vi "Sort Particle Reports.vi"(1 "Report 2":T1, 2 "Report 1":T1) -> (0 "x > y?":bool)   [LabVIEW 2025]
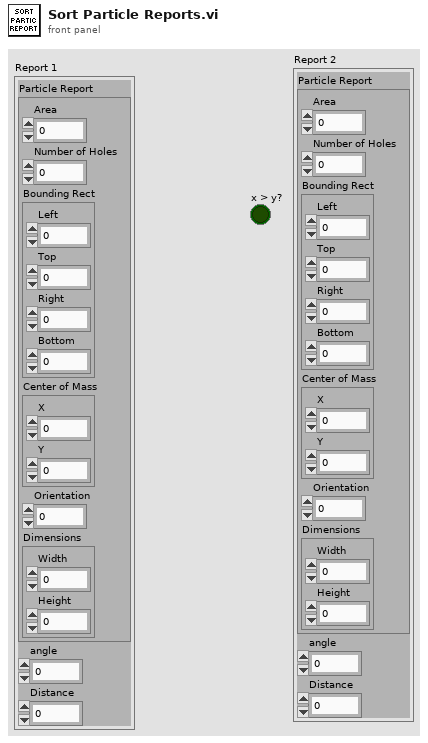
[diagram p1: front panel]
types:
  T1 = cluster{"Particle Report":cluster{"Area":dbl, "Number of Holes":dbl, "Bounding Rect":cluster{"Left":dbl, "Top":dbl, "Right":dbl, "Bottom":dbl}, "Center of Mass":cluster{"X":dbl, "Y":dbl}, "Orientation":dbl, "Dimensions":cluster{"Width":dbl, "Height":dbl}}, "angle":dbl, "Distance":ext}
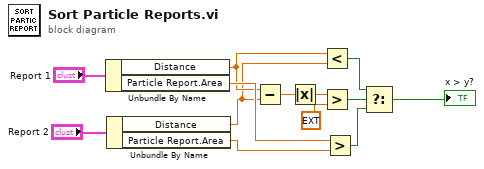
[diagram p0: block diagram]
diagram:
  n1 = Unbundle By Name("Report 1") -> ("Distance"=w3:ext, "Particle Report.Area"=w6:dbl)
  n2 = Unbundle By Name("Report 2") -> ("Distance"=w2:ext, "Particle Report.Area"=w5:dbl)
  n3 = Subtract(x=w3, y=w2) -> (x-y=w12:ext)
  n4 = Absolute Value(x=w12) -> (abs(x)=w4:ext)
  n5 = Less?(x=w3, y=w2) -> (x < y?=w1:bool)
  n6 = Greater?(x=w4, y=ext 2.0) -> (0:w11:bool)
  n7 = Greater?(x=w6, y=w5) -> (0:w7:bool)
  n8 = Select(t=w1, s=w11, f=w7) -> (s? t:f=→"x > y?":bool)
